vi "Add Attribute.vi"(4 "Private?":bool, 5 "Update Pointer?":bool, 6 "Pointer?":bool, 7 "ID":string, 8 "error in (no error)":errorcluster, 9 "Attribute":variant, 10 "Attribute Name":string, 11 "Test Executive in":refnum<class "Test Executive.lvclass">) -> (0 "error out":errorcluster, 1 "Replaced?":bool, 2 "Attribute ID out":string, 3 "Test Executive out":refnum<class "Test Executive.lvclass">)   [LabVIEW 2020, in "Test Executive.lvlib" / "Test Executive.lvclass"]
uses:
  <vilib>/gpm_packages/@cs/test-executive/Source/Test Executive/TestExecutive/Test Executive.lvclass
  <vilib>/gpm_packages/@cs/test-executive/Source/Test Executive/TestExecutive/Test Executive.lvclass/Test Executive.ctl
  96bffb70-7b20-4873-bea8-60f34433eb5c.vi
  <vilib>/gpm_packages/@cs/linked-list/Source/Linked List/ILinkedList/ILinked List.lvclass
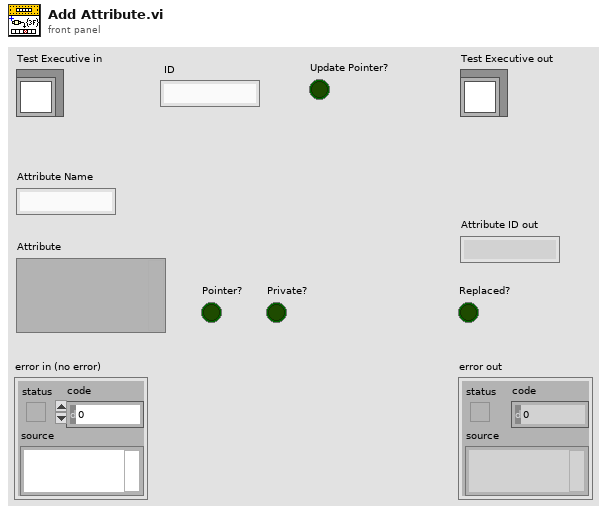
[diagram p1: front panel]
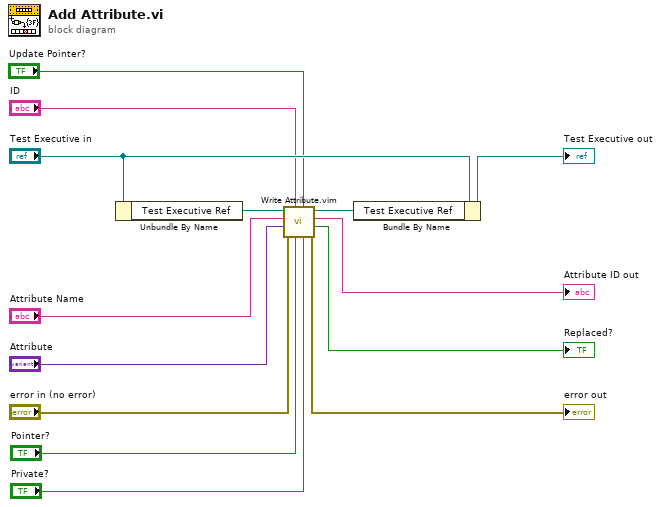
[diagram p0: block diagram]
diagram:
  n1 = Unbundle By Name("Test Executive in") -> ("Test Executive Ref"=w14:refnum<data-value>)
  n2 = call "Write Attribute.vim"("Private?"="Private?", "Update Pointer?"="Update Pointer?", "Pointer?"="Pointer?", "Linked List ID"="ID", "error in (no error)"="error in (no error)", "Attribute"="Attribute", "Attribute Name"="Attribute Name", "Linked List Ref"=w14) -> ("error out"=→"error out":errorcluster, "Replaced?"=→"Replaced?":bool, "Attribute ID out"=→"Attribute ID out":string, "Linked List Ref out"=w11:refnum<data-value>)
  n3 = Bundle By Name(cluster="Test Executive in", "Test Executive Ref"=w11) -> (→"Test Executive out":refnum<class "Test Executive.lvclass">)
